vi "Main - Manual Active FGV.vi"(7 "Action":T1=enum."Write", 8 "error In":errorcluster, 9 "Timer":dbl format="%#_13g", 10 "Use Timer?":bool, 11 "Manual? In":bool) -> (0 "error out":errorcluster, 1 "Timer out":dbl, 2 "Use Timer? out":bool, 3 "Manual? Out":bool)   [LabVIEW 2019]
uses:
  Controls/FGV States.ctl
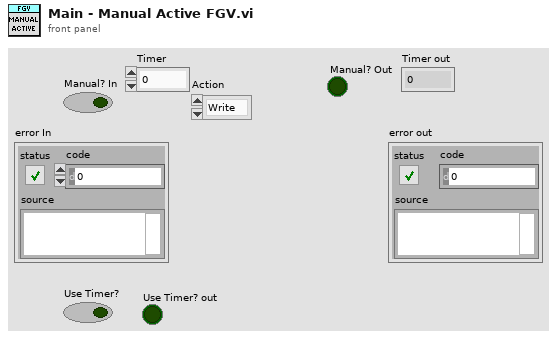
[diagram p1: front panel]
types:
  T1 = typedef "FGV States.ctl" = enum16{"Read", "Write"}
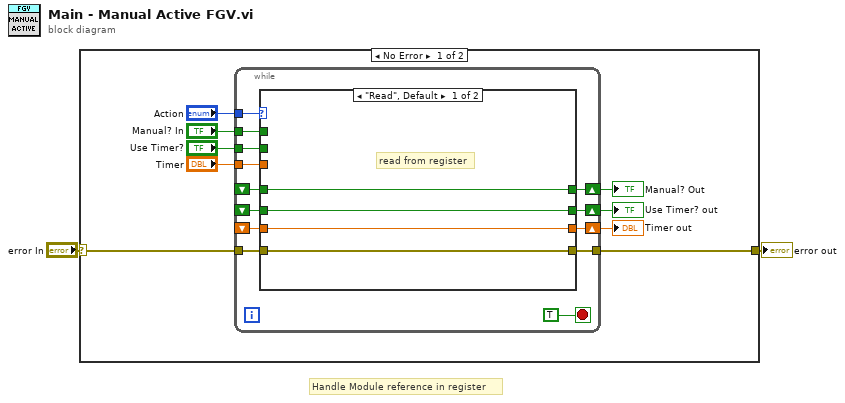
[diagram p0: block diagram]
diagram:
  # "Handle Module reference in register"
  n1 = case shown="No Error" "error In" {
    selector: "error In" -> [w10 w33]
    tunnel: [w9 w33] -> w1
    frame No Error {
      n2 = while {
        tunnel: "Action" -> [w24]
        tunnel: "Manual? In" -> [w21]
        shift-right: [w22] -> w7
        shift-left: _ -> [w20]
        tunnel: [w19] -> w9
        tunnel: w10 -> [w18]
        tunnel: "Use Timer?" -> [w17]
        shift-right: [w16] -> w5
        shift-left: _ -> [w15]
        tunnel: "Timer" -> [w13]
        shift-right: [w14] -> w3
        shift-left: _ -> [w12]
        stop <- TRUE stop-if-true
        n3 = case shown="\"Read\", Default" w24 {
          tunnel: [w27 w32] -> w22
          tunnel: w21 -> [_ w32]
          tunnel: w20 -> [w27 _]
          tunnel: [w28 w31] -> w19
          tunnel: w18 -> [w28 w31]
          tunnel: w17 -> [_ w30]
          tunnel: [w26 w30] -> w16
          tunnel: w15 -> [w26 _]
          tunnel: [w25 w29] -> w14
          tunnel: w13 -> [_ w29]
          tunnel: w12 -> [w25 _]
          frame "Read", Default {
            # "read from register"
          }
          frame "Write" {
            # "write to register"
          }
        }
      }
      "Manual? Out" <- w7
      "Use Timer? out" <- w5
      "Timer out" <- w3
    }
    frame Error {
    }
  }
  "error out" <- w1
